vi "Main.vi"() -> ()   [LabVIEW 2016]
doc: "Main controller to read from an EK-P4 board connected to a squeezable ball, detect squeeze and release, and send it over a TCP connection to a waiting client (in this case the Matlab experiment). Choose the data file name, port and measurment interval and press start to start acquiring data. Close window to exit.\n\nSaves all data to basename_subject_id_date_time. last row in file (time = -1111) are the thresholds used.\n\ndiagram structure\n-------------------\nevent loop: start acquisition and close window.\nhardware loop: initialize, acquire data, close. all data is sent to data analysis loop\ndata analysis loop: display, save, analyze, send and receive from TCP.\nTCP loop (TCP Kernel): TCP server, sends and receives over port 55555"
uses:
  command_cluster.ctl
  data_command_enum.ctl
  HW loop state.ctl
  LoopData.ctl
  EK-P4/EK-P4.lvclass
  DataType.ctl
  FileData.ctl
  range_cluster.ctl
  EK-P4 Global.vi
  <vilib>/Utility/file.llb/Write Delimited Spreadsheet (string).vi
  <vilib>/Utility/config.llb/Read Key (Path).vi
  <vilib>/Utility/config.llb/Write Key (Path).vi
  <vilib>/Analysis/NI_AALPro.lvlib
  <vilib>/Utility/config.llb/NI_LVConfig.lvlib
panel:
  in  "Record\nTime":u16
  out "# elements in queue":i32
  in  "minimum":dbl=20.0 caption="Measurement interval [ms]"
  in  "Squeeze 2":bool
  in  "Release 2":bool
  out "strong \nrelease threshold":dbl
  out "strong\nsqueeze threshold":dbl
  out "releases 2":u16
  out "squeezes 2":u16
  out "release 2":bool
  out "squeeze 2":bool
  out "size(s) 2":i32
  out "size(s)":i32
  in  "COM port 2":refnum<visa-resource-name> caption="COM port"
  in  "COM port 1":refnum<visa-resource-name> caption="COM port"
  in  "Subject Id":string
  in  "Base File Name":string
  in  "Folder to save to":path
  in  "Release":bool
  in  "Squeeze":bool
  out "error out":errorcluster
  in  "Start":bool
  out "release":bool
  out "squeeze":bool
  in  "threshold squeeze (Pa)":dbl=100.0 caption="Measurement interval [ms]"
  in  "width (pixels)":u16=20 caption="Measurement interval [ms]"
  in  "threshold release (Pa)":dbl=-100.0 caption="Measurement interval [ms]"
  out "squeezes":u16
  out "releases":u16
  in  "Measurement interval [ms]":u16=2 min=2 step=1
  out "data string":string
  out "error  out":errorcluster
  out "Data flow/dp":dbl[][](graph) caption="Waveform Graph"
  out "integral":dbl[][](graph) caption="Waveform Graph"
  out "Status":string
  # "Measurement parameters"
  # "Squeeze-release"
  # "Testing & debug"
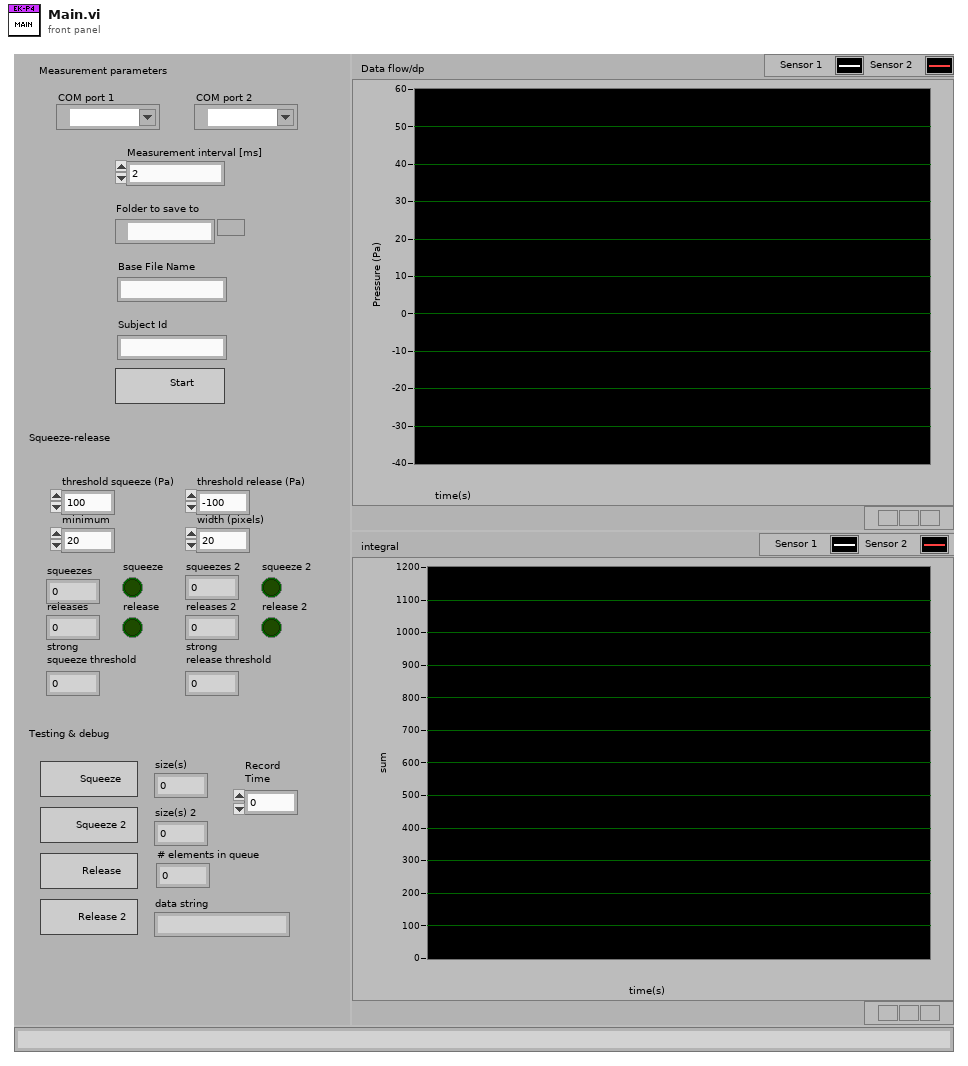
[diagram p1: front panel]
types:
  T1 = typedef "DataType.ctl" = cluster{"command":T2, "data":variant}
  T2 = typedef "data_command_enum.ctl" = enum16{"data", "display", "quit", "save", "filepath", "weak left", "state", "weak right", "strong left", "strong right", "stopRecording", "close", "sid"}
  T3 = typedef "LoopData.ctl" = cluster{"Hardware":refnum<class "EK-P4.lvclass">, "Hardware 2":refnum<class "EK-P4.lvclass">, "startTime":timestamp}
  T4 = typedef "HW loop state.ctl" = enum16{"Init", "Start", "Read", "Close", "Error", "Idle", "Exit", "Close and Exit"}
  T5 = typedef "command_cluster.ctl" = cluster{"command":T2}
  T6 = typedef "NI_LVConfig.lvlib/Config Data RefNum.ctl" = refnum<k1>
  T7 = enum16{"open", "replace", "create", "open or create", "replace or create", "replace or create with confirmation"}
  T8 = typedef "DataLoopCluster.ctl" = cluster{"all data 1":dbl[], "all data 2":dbl[], "data chunk 1":dbl[], "data chunk 2":dbl[], "number of squeezes":u16, "number of releases":u16, "Time(ms)":i64, "startWeak":timestamp, "startTime":timestamp, "Filepath":path, "time interval":u16, "recording":bool, "recording data":dbl[], "number of squeezes 2":u16, "number of releases 2":u16, "Signal":T9, "All State":string[], "Experiment State":string, "all detect state":string[], "detect State":string, "Ranges":cluster{"Strong Left":T10, "Strong Right":T10, "Weak Left":T10, "Weak Right":T10}, "ball 1":timestamp, "ball 2":timestamp, "RecordTime":u16}
  T9 = typedef "SignalType.ctl" = enum16{"weak left", "weak right", "strong left", "strong right"}
  T10 = typedef "range_cluster.ctl" = cluster{"Max":dbl, "Min":dbl}
  T11 = typedef "FileData.ctl" = cluster{"appended path":path, "Measurement interval [ms]":u16}
  T12 = enum32{"invalid app kind", "Development System", "Run Time System", "Student Edition", "Embedded LabVIEW", "Evaluation", "Custom"}
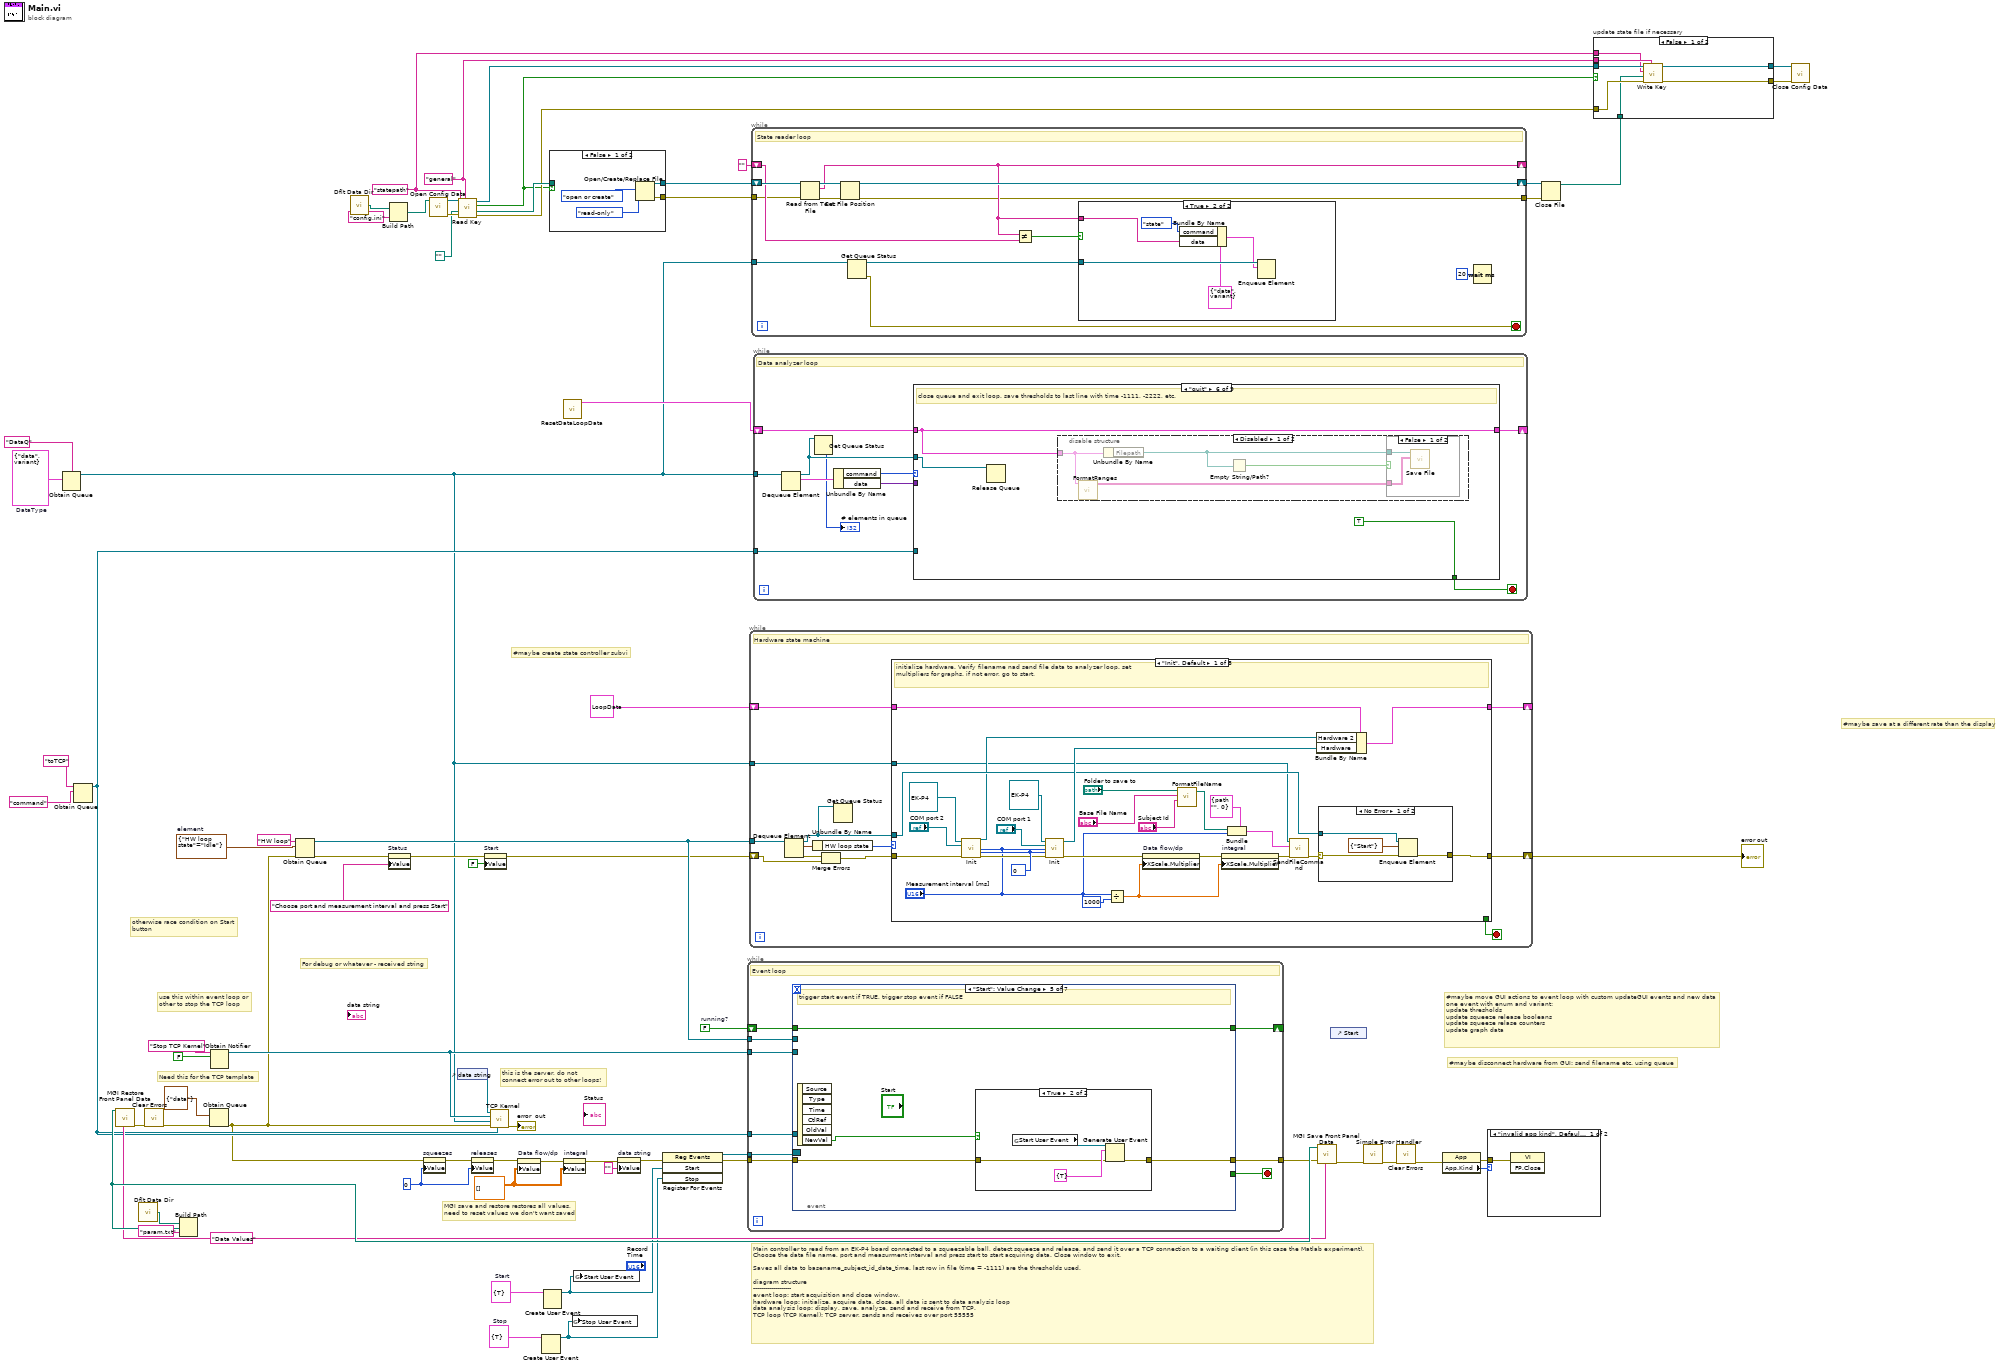
[diagram p0: block diagram]
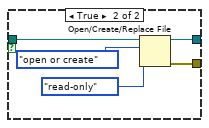
[diagram p2: hidden frame]
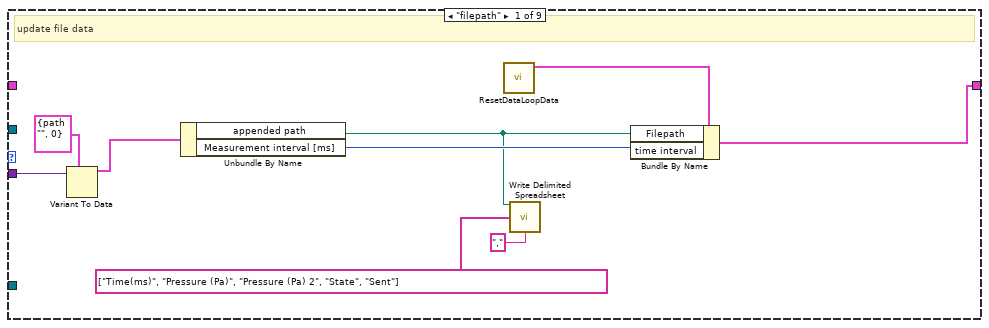
[diagram p5: hidden frame]
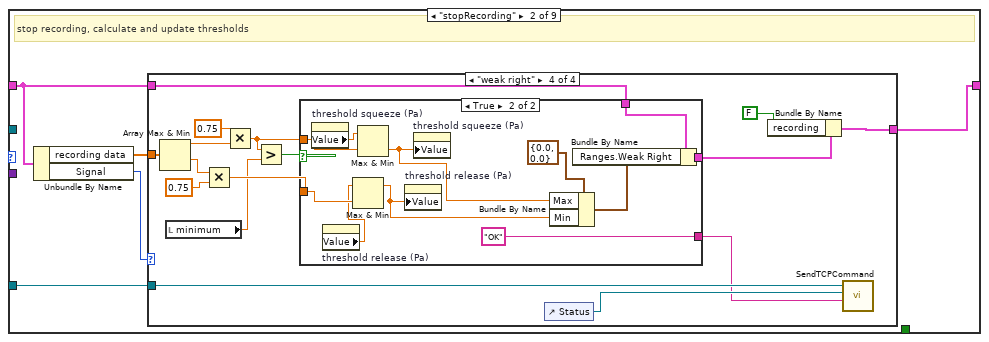
[diagram p6: hidden frame]
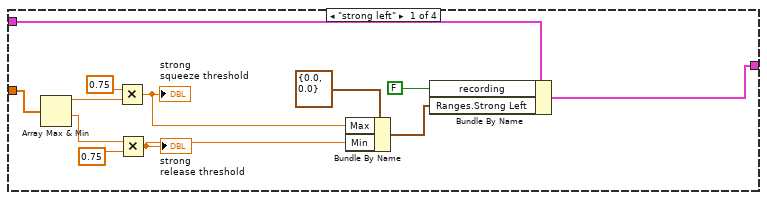
[diagram p7: hidden frame]
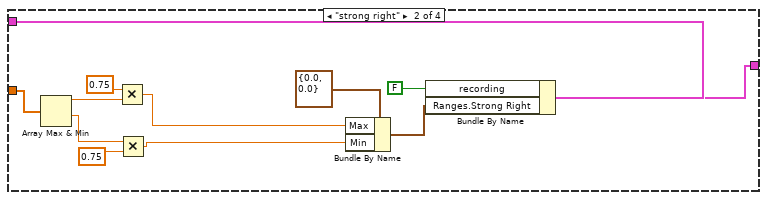
[diagram p8: hidden frame]
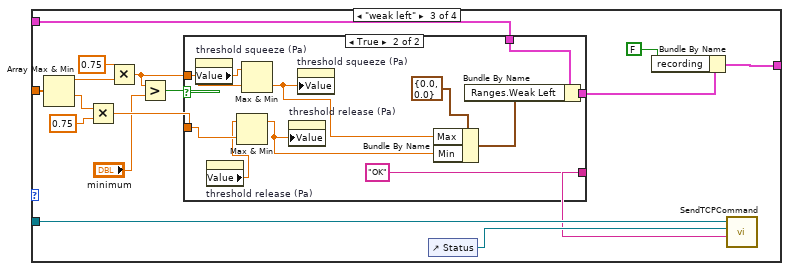
[diagram p9: hidden frame]
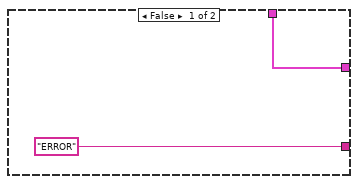
[diagram p10: hidden frame]
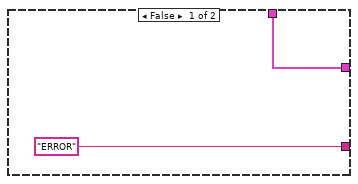
[diagram p11: hidden frame]
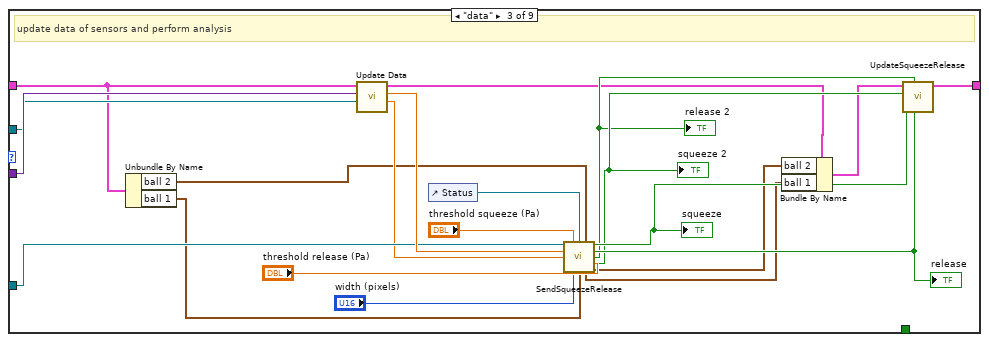
[diagram p12: hidden frame]
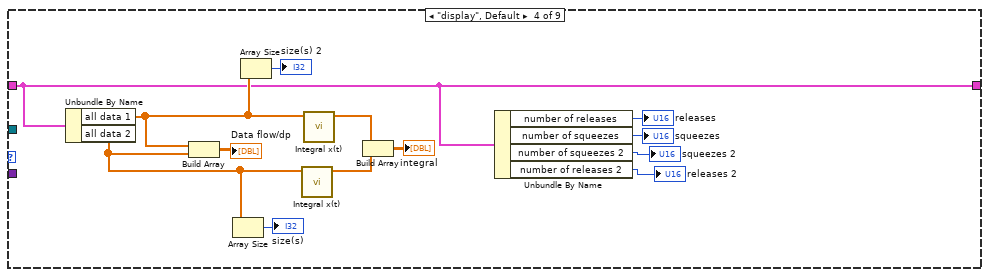
[diagram p13: hidden frame]
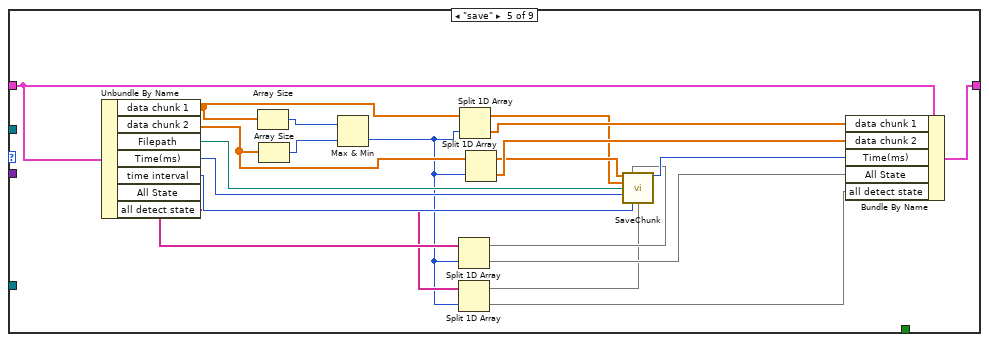
[diagram p14: hidden frame]
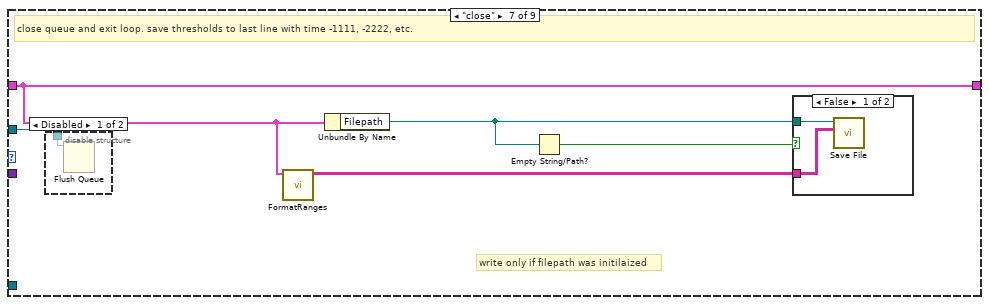
[diagram p17: hidden frame]
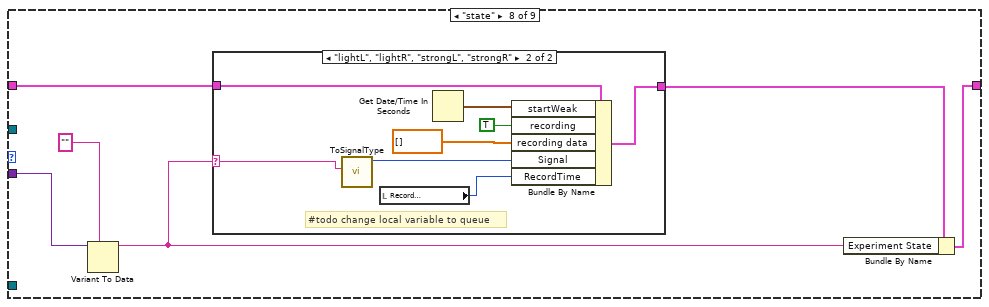
[diagram p20: hidden frame]
diagram:
  w8 = "general" ("section")
  w7 = "statepath" ("key")
  w26 = FALSE  # running?
  w28 = cluster{"Stop":bool} {"Stop"=TRUE}  # Stop
  w32 = cluster{"Start":bool} {"Start"=TRUE}  # Start
  w41 = T1 {"command"=enum."data", "data"=variant(dbl[] [])}  # DataType
  w39 = dbl[][] [] ("Data flow/dp")
  w43 = u16 0 ("squeezes")
  w49 = "Data Values" ("Section Name (\"Data Values\")")
  w62 = cluster{"HW loop state":T4} {"HW loop state"=enum."Idle"}  # element
  # "#maybe create state controller subvi"
  # "otherwise race condition on Start\nbutton"
  # "Main controller to read from an EK-P4 board connected to a squeezable ball, detect squeeze and release, and send it over a TCP connection to a waiting client (in this case the Matlab experiment). \nChoose the data file name, port and measurment interval and press start to start acquiring data. Close window to exit.\n\nSaves all data to basename_subject_id_date_time. last row in file (time = -1111) are the thresholds used.\n\ndiagram structure\n-------------------\nevent loop: start acquisition and close window.\nhardware loop: initialize, acquire data, close. all data is sent to data analysis loop\ndata analysis loop: display, save, analyze, send and receive from TCP.\nTCP loop (TCP Kernel): TCP server, sends and receives over port 55555"
  # "#maybe disconnect hardware from GUI: send filename etc. using queue"
  # "#maybe save at a different rate than the display"
  # "MGI save and restore restores all values,\nneed to reset values we don't want saved"
  # "#maybe move GUI actions to event loop with custom updateGUI events and new data\none event with enum and variant:\nupdate thresholds\nupdate squeeze release booleans\nupdate squeeze relase counters\nupdate graph data"
  # "this is the server, do not\nconnect error out to other loops!"
  # "For debug or whatever - received string"
  # "use this within event loop or \nother to stop the TCP loop"
  # "Need this for the TCP template"
  n1 = Obtain Queue(name (unnamed)="DataQ", element data type=w41) -> (queue out=w21:refnum<queue>)  [unwired: 3 in, 2 out]
  n2 = Obtain Queue(name (unnamed)="toTCP", element data type="command" ("name (unnamed)")) -> (queue out=w36:refnum<queue>)  [unwired: 3 in, 2 out]
  n3 = call <vilib>:"Dflt Data Dir.vi"() -> ("App:Default Data Directory"=w23:path)
  n4 = Build Path(base path=w23, name or relative path="param.txt") -> (appended path=w50:path)
  n5 = call <userlib>:"MGI Restore Front Panel Data.vi"("Section Name (\"Data Values\")"=w49, "Path"=w50) -> ("Error Out"=w48:errorcluster)  [unwired: 9 in]
  n6 = call <vilib>:"Clear Errors.vi"("error in (no error)"=w48) -> ("error out"=w47:errorcluster)  [unwired: 5 in, 1 out]
  n7 = Obtain Queue(element data type=T5 {"command"=enum."data"} ("chair_command_cluster"), error in (no error)=w47) -> (error out=w22:errorcluster)  [unwired: 3 in, 2 out]
  n8 = Obtain Notifier(name (unnamed)="Stop TCP Kernel", notification data type=FALSE) -> (notifier out=w64:refnum<notifier>)  [unwired: 2 in, 2 out]
  n9 = Obtain Queue(name (unnamed)="HW loop", element data type=w62, error in (no error)=w22) -> (queue out=w61:refnum<queue>, error out=w60:errorcluster)  [unwired: 2 in, 1 out]
  n10 = call <vilib>:"Dflt Data Dir.vi"() -> ("App:Default Data Directory"=w2:path)
  n11 = property on="Status" class="Str"(error in=w60, "Value"="Choose port and measurement interval and press Start" ("Status")) -> (error out=w55:errorcluster)  [unwired: 1 in, 1 out]
  n12 = Build Path(base path=w2, name or relative path="config.ini") -> (appended path=w11:path)
  n13 = property on="squeezes" class="DigNum (strict)"(error in=w22, "Value"=w43) -> (error out=w46:errorcluster)  [unwired: 1 in, 1 out]
  n14 = call <vilib>:"Open Config Data.vi"("configuration file path"=w11) -> ("error out"=w15:errorcluster, "refnum"=w14:T6)  [unwired: 8 in, 1 out]
  n15 = control-ref of="data string"() -> (w66:refnum<vi>)
  n16 = call-poly <vilib>:"Read Key.vi"("section"=w8, "error in (no error)"=w15, "default value"=path "", "key"=w7, "refnum"=w14) -> ("error out"=w6:errorcluster, "value"=w10:path, "found?"=w1:bool, "refnum out"=w9:T6)  [unwired: 3 in]
  n17 = property on="releases" class="DigNum (strict)"(error in=w46, "Value"=w43) -> (error out=w45:errorcluster)  [unwired: 1 in, 1 out]
  n18 = property on="Start" class="Bool (strict)"(error in=w55, "Value"=FALSE ("Visible")) -> (error out=w57:errorcluster)  [unwired: 1 in, 1 out]
  n19 = call "TCP Kernel.vi"("HW queue in"=w36, "error in (no error)"=w22, "queue in"=w21, "Stop Kernel Notifier"=w64, "Data indicator"=w66) -> ("error out"=→"error  out":errorcluster)  [unwired: 6 in]
  n20 = property on="Data flow/dp" class="WFGraph (strict)"(error in=w45, "Value"=w39) -> (error out=w44:errorcluster)  [unwired: 1 in, 1 out]
  n21 = Create User Event(user event datatype=w28) -> (user event=w27:refnum<user-event>)  [unwired: 1 in, 1 out]
  n22 = Create User Event(user event datatype=w32) -> (user event=w30:refnum<user-event>)  [unwired: 1 in, 1 out]
  n23 = case shown="False" w1 {
    tunnel: [w73 w80] -> w20
    tunnel: [w72 w79] -> w17
    tunnel: w10 -> [_ w76]
    frame False {
      n24 = Open/Create/Replace File(operation (0:open)=T7."open or create", access (0:read/write)=enum16{"read/write", "read-only", "write-only"}."read-only") -> (refnum out=w73:refnum<file>, error out=w72:errorcluster)  [unwired: 4 in, 1 out]
    }
    frame True {
      n25 = Open/Create/Replace File(file path (use dialog)=w76, operation (0:open)=T7."open or create", access (0:read/write)=enum16{"read/write", "read-only", "write-only"}."read-only") -> (refnum out=w80:refnum<file>, error out=w79:errorcluster)  [unwired: 3 in, 1 out]
    }
  }
  n26 = call "ResetDataLoopData.vi"() -> ("cluster"=w40:T8)  [unwired: 11 in]
  n27 = property on="integral" class="WFGraph (strict)"(error in=w44, "Value"=w39) -> (error out=w35:errorcluster)  [unwired: 1 in, 1 out]
  n28 = global write "EK-P4 Global.vi" "Stop User Event"(w27) -> ()
  n29 = global write "EK-P4 Global.vi" "Start User Event"(w30) -> ()
  n30 = property on="data string" class="Str"(error in=w35, "Value"="" ("data string")) -> (error out=w34:errorcluster)  [unwired: 1 in, 1 out]
  n31 = register-events(error in=w34, w30, w27) -> (reference out=w29:refnum<event-registration>, error out=w31:errorcluster)  [unwired: 1 in]
  n32 = while "Event loop" {
    tunnel: w64 -> [w89]
    tunnel: w31 -> [w87]
    tunnel: w61 -> [w86]
    tunnel: w36 -> [w85]
    tunnel: [w84] -> w38
    tunnel: w29 -> [w83]
    shift-right: [w81] -> _
    shift-left: w26 -> [w82]
    stop <- w88 stop-if-true
    # "Event loop"
    n33 = event shown="[4] \"Start\": Value Change" {
      selector: w83 -> [_ _ _ _ _ _ _]
      dyn-events: _ -> [_ _ _ _ _ _ _]
      timeout: _ -> [_ _ _ _ _ _ _]
      tunnel: w89 -> [_ w100 _ _ _ _ _]
      tunnel: [_ w98 _ _ _ _ _] -> w88
      tunnel: w87 -> [w91 w96 w103 w128 w146 w157 w167]
      tunnel: w86 -> [_ w97 w108 w129 _ _ _]
      tunnel: w85 -> [_ _ _ w127 _ w159 w169]
      tunnel: [w91 w96 w102 w128 w145 w157 w167] -> w84
      tunnel: w82 -> [w90 w95 w107 w126 w147 w156 w166]
      tunnel: [w90 w95 w106 w125 w147 w156 w166] -> w81
      event Timeout {
        n34 = event-data() -> ()  [unwired: 1 in, 3 out]
      }
      event Panel Close? {
        w98 = TRUE ("Discard?")
        # "exit TCP and hardware loops. If running, close and exit, otherwise exit"
        n35 = event-data() -> ()  [unwired: 1 in, 4 out]
        n36 = Send Notification(notification=TRUE, notifier=w100) -> ()  [unwired: 1 in, 2 out]
        n37 = Select(t=cluster{"HW loop state":T4} {"HW loop state"=enum."Close and Exit"}, s=w95, f=cluster{"HW loop state":T4} {"HW loop state"=enum."Exit"} ("element")) -> (s? t:f=w93:cluster{"HW loop state":T4})
        n38 = Enqueue Element(queue=w97, element=w93) -> ()  [unwired: 2 in, 3 out]
        n39 = event-data("Discard?"=w98) -> ()  [unwired: 1 in, 1 out]
      }
      event User Event {
        # "if sent with FALSE, trigger start"
        # "stop hardware acquisition and go to idle state"
        n40 = event-data() -> ("Stop"=w105:bool)  [unwired: 1 in]
        n41 = case shown="True" w107 {
          tunnel: w108 -> [_ w124]
          tunnel: [w116 FALSE ("running?")] -> w106
          tunnel: [w115 w118] -> w104
          tunnel: w103 -> [w115 w117]
          frame False {
            w116 = FALSE  # running?
          }
          frame True {
            # "go to idle state"
            n42 = control-ref of="Start"() -> (w121:refnum<vi>)
            n43 = Enqueue Element(queue=w124, element=cluster{"HW loop state":T4} {"HW loop state"=enum."Close"}, error in (no error)=w117) -> (error out=w119:errorcluster)  [unwired: 1 in, 2 out]
            n44 = property class="Bool (strict)"(reference=w121, error in=w119, "Visible"=TRUE) -> (error out=w118:errorcluster)  [unwired: 1 out]
          }
        }
        n45 = property on="Start" class="Bool (strict)"("Value"=FALSE ("Start")) -> ()  [unwired: 2 in, 2 out]
        n46 = case shown="False" w105 {
          tunnel: w104 -> [w111 w114]
          tunnel: [w110 w114] -> w102
          frame False {
            # "wait, otherwise flushes init\non close"
            n47 = global read "EK-P4 Global.vi" "Start User Event"() -> (w113:refnum<user-event>)
            n48 = Wait (ms)(milliseconds to wait=u32 500) -> ()  [unwired: 1 out]
            n49 = Generate User Event(user event=w113, event data cluster=cluster{bool} {TRUE} ("event data"), error in=w111) -> (error out=w110:errorcluster)  [unwired: 1 in, 1 out]
          }
          frame True {
          }
        }
      }
      event User Event {
        # "Start acquiring hardware data"
        n50 = event-data() -> ()  [unwired: 1 in, 5 out]
        n51 = case shown="False" w126 {
          selector: w126 -> [_ w142]
          tunnel: w129 -> [w135 _]
          tunnel: w127 -> [w132 _]
          tunnel: [TRUE ("running?") w142] -> w125
          frame False {
            # "not running - start as usual"
            n52 = disable-structure shown="Disabled" {
              disable-tunnel: w132 -> [w139 _]
              frame Disabled {
                n53 = local read "Subject Id"() -> (w137:string)
                n54 = control-ref of="Status"() -> (w140:refnum<vi>)
                n55 = Concatenate Strings("SID: " ("format string"), w137) -> (w136:string)
                n56 = call "SendTCPCommand.vi"("Command"=w136, "Status"=w140, "queue in"=w139) -> ()  [unwired: 7 in, 2 out]
              }
              frame Enabled {
              }
            }
            n57 = Enqueue Element(queue=w135, element=cluster{"HW loop state":T4} {"HW loop state"=enum."Init"}) -> ()  [unwired: 2 in, 3 out]
            n58 = property on="Status" class="Str"("Value"="Receiving data. Close window to Exit" ("Status")) -> ()  [unwired: 2 in, 2 out]
            n59 = property on="Start" class="Bool (strict)"("Value"=TRUE ("Start")) -> ()  [unwired: 2 in, 2 out]
          }
          frame True {
            # "send with false, will trigger start"
            # "already running - \nstop and start again"
            n60 = global read "EK-P4 Global.vi" "Stop User Event"() -> (w143:refnum<user-event>)
            n61 = Generate User Event(user event=w143, event data cluster=cluster{bool} {FALSE} ("event data")) -> ()  [unwired: 2 in, 2 out]
          }
        }
      }
      event "Start": Value Change {
        # "trigger start event if TRUE, trigger stop event if FALSE"
        n62 = event-data() -> ("NewVal"=w144:bool)  [unwired: 1 in, 5 out]
        n63 = case shown="True" w144 {
          tunnel: w146 -> [w149 w153]
          tunnel: [w148 w152] -> w145
          frame False {
            n64 = global read "EK-P4 Global.vi" "Stop User Event"() -> (w151:refnum<user-event>)
            n65 = Generate User Event(user event=w151, event data cluster=cluster{bool} {TRUE} ("event data"), error in=w149) -> (error out=w148:errorcluster)  [unwired: 1 in, 1 out]
          }
          frame True {
            n66 = global read "EK-P4 Global.vi" "Start User Event"() -> (w155:refnum<user-event>)
            n67 = Generate User Event(user event=w155, event data cluster=cluster{bool} {TRUE} ("event data"), error in=w153) -> (error out=w152:errorcluster)  [unwired: 1 in, 1 out]
          }
        }
      }
      event "Squeeze", "Release": Value Change {
        # "for debug, send squeeze or release over TCP"
        n68 = event-data() -> ("CtlRef"=w164:refnum<vi>)  [unwired: 1 in]
        n69 = control-ref of="Squeeze"() -> (w165:refnum<vi>)
        n70 = Equal?(x=w165, y=w164) -> (x = y?=w163:bool)
        n71 = control-ref of="Status"() -> (w158:refnum<vi>)
        n72 = Select(t="s1" ("element"), s=w163, f="r1" ("element")) -> (s? t:f=w160:string)
        n73 = call "SendTCPCommand.vi"("Command"=w160, "Status"=w158, "queue in"=w159) -> ()  [unwired: 7 in, 2 out]
      }
      event "Release 2", "Squeeze 2": Value Change {
        # "for debug, send squeeze or release over TCP"
        n74 = event-data() -> ("CtlRef"=w174:refnum<vi>)  [unwired: 1 in, 1 out]
        n75 = control-ref of="Squeeze 2"() -> (w175:refnum<vi>)
        n76 = Equal?(x=w175, y=w174) -> (x = y?=w173:bool)
        n77 = control-ref of="Status"() -> (w168:refnum<vi>)
        n78 = Select(t="s2" ("element"), s=w173, f="r2" ("element")) -> (s? t:f=w170:string)
        n79 = call "SendTCPCommand.vi"("Command"=w170, "Status"=w168, "queue in"=w169) -> ()  [unwired: 7 in, 2 out]
      }
    }
  }
  n80 = while {
    tunnel: w61 -> [w187]
    shift-right: [w183] -> _
    shift-left: T3 {"Hardware"=refnum, "Hardware 2"=refnum, "startTime"=timestamp(0 s since 1904-01-01)} ("output cluster") -> [w184]
    shift-right: [w180] -> w59
    shift-left: w57 -> [w178]
    tunnel: w21 -> [w177]
    stop <- w181 stop-if-true
    # "Hardware state machine"
    n81 = Dequeue Element(queue=w187) -> (queue out=w176:refnum<queue>, element=w186:cluster{"HW loop state":T4}, error out=w182:errorcluster)  [unwired: 2 in, 1 out]
    n82 = Unbundle By Name(w186) -> ("HW loop state"=w185:T4)
    n83 = Merge Errors(w182, w178) -> (w179:errorcluster)
    n84 = Get Queue Status(queue=w176) -> ()  [unwired: 2 in, 8 out]
    n85 = case shown="\"Init\", Default" w185 {
      tunnel: w184 -> [w205 w231 w259 w288 w303 w312 w323 w330]
      tunnel: [w213 w230 w259 w288 w303 w312 w323 w330] -> w183
      tunnel: w176 -> [w206 w225 w260 w279 _ _ w319 w328]
      tunnel: w179 -> [w198 w235 w263 w285 w301 w309 w322 w329]
      tunnel: [w207 w227 w261 w280 w301 w305 w316 w325] -> w180
      tunnel: [_ _ _ FALSE TRUE TRUE _ _] -> w181
      tunnel: w177 -> [w195 _ w257 w282 w300 w306 _ _]
      frame "Init", Default {
        w200 = u8 0 ("address (USB SensorCable) 2")
        # "initialize hardware. Verify filename nad send file data to analyzer loop. set\nmultipliers for graphs. if not error, go to start."
        n86 = call-dynamic "Init.vi"("EK-P4.lvclass"=refnum<class "EK-P4.lvclass"> refnum, "VISA Refnum in"="COM port 2", "Measurement interval [ms] in"="Measurement interval [ms]", "address (USB SensorCable)"=w200, "error in (no error)"=w198) -> ("EK-P4.lvclass 2"=w199:refnum<class "EK-P4.lvclass">, "error out"=w197:errorcluster)  [unwired: 8 in, 1 out]
        n87 = call-dynamic "Init.vi"("EK-P4.lvclass"=refnum<class "EK-P4.lvclass"> refnum, "VISA Refnum in"="COM port 1", "Measurement interval [ms] in"="Measurement interval [ms]", "address (USB SensorCable)"=w200, "error in (no error)"=w197) -> ("EK-P4.lvclass 2"=w209:refnum<class "EK-P4.lvclass">, "error out"=w196:errorcluster)  [unwired: 8 in, 1 out]
        n88 = Divide(x="Measurement interval [ms]", y=u16 1000) -> (x/y=w211:dbl)
        n89 = property on="Data flow/dp" class="WFGraph (strict)"(error in=w196, "XScale.Multiplier"=w211) -> (error out=w208:errorcluster)  [unwired: 1 in, 1 out]
        n90 = call "FormatFileName.vi"("Subject Id"="Subject Id", "Base file Name"="Base File Name", "Folder to save to"="Folder to save to") -> ("appended path"=w192:path)  [unwired: 8 in]
        n91 = property on="integral" class="WFGraph (strict)"(error in=w208, "XScale.Multiplier"=w211) -> (error out=w194:errorcluster)  [unwired: 1 in, 1 out]
        n92 = Bundle(cluster=T11 {"appended path"=path "", "Measurement interval [ms]"=0}, "appended path"=w192, "Measurement interval [ms]"="Measurement interval [ms]") -> (w190:T11)
        n93 = call "SendFileCommand.vi"("error in (no error)"=w194, "file data"=w190, "Queue in"=w195) -> ("error out"=w193:errorcluster)  [unwired: 7 in, 1 out]
        n94 = Bundle By Name(cluster=w205, "Hardware 2"=w199, "Hardware"=w209) -> (w213:T3)
        n95 = case shown="No Error" w193 {
          selector: w193 -> [w217 w219]
          tunnel: [w216 w221] -> w207
          tunnel: w206 -> [w215 w222]
          frame No Error {
            n96 = Enqueue Element(queue=w215, element=cluster{"HW loop state":T4} {"HW loop state"=enum."Start"}, error in (no error)=w217) -> (error out=w216:errorcluster)  [unwired: 1 in, 2 out]
          }
          frame Error {
            n97 = Enqueue Element(queue=w222, element=cluster{"HW loop state":T4} {"HW loop state"=enum."Error"}) -> (error out=w220:errorcluster)  [unwired: 2 in, 2 out]
            n98 = Merge Errors(w220, w219) -> (w221:errorcluster)
          }
        }
      }
      frame "Start" {
        # "if not error go to read"
        # "start measurement in each sensor. Becasue they can't be started exactly simulataneously, the sensors have a small phase difference. this is ignored in the file and everywhere else. save start time for timing of display and save commands"
        n99 = Unbundle By Name(w231) -> ("Hardware 2"=w232:refnum<class "EK-P4.lvclass">, "Hardware"=w233:refnum<class "EK-P4.lvclass">)
        n100 = call-dynamic "Start Measurement.vi"("EK-P4.lvclass"=w233, "error in (no error)"=w235) -> ("EK-P4.lvclass 2"=w228:refnum<class "EK-P4.lvclass">, "error out"=w234:errorcluster)  [unwired: 12 in]
        n101 = call-dynamic "Start Measurement.vi"("EK-P4.lvclass"=w232, "error in (no error)"=w234) -> ("EK-P4.lvclass 2"=w229:refnum<class "EK-P4.lvclass">, "error out"=w226:errorcluster)  [unwired: 12 in]
        n102 = Get Date/Time In Seconds() -> (seconds since 1Jan1904=w224:timestamp)
        n103 = case shown="No Error" w226 {
          selector: w226 -> [w238 w240]
          tunnel: [w237 w242] -> w227
          tunnel: w225 -> [w236 w243]
          frame No Error {
            n104 = Enqueue Element(queue=w236, element=cluster{"HW loop state":T4} {"HW loop state"=enum."Read"}, error in (no error)=w238) -> (error out=w237:errorcluster)  [unwired: 1 in, 2 out]
          }
          frame Error {
            n105 = Enqueue Element(queue=w243, element=cluster{"HW loop state":T4} {"HW loop state"=enum."Error"}) -> (error out=w241:errorcluster)  [unwired: 2 in, 2 out]
            n106 = Merge Errors(w241, w240) -> (w242:errorcluster)
          }
        }
        n107 = Bundle By Name(cluster=w231, "Hardware 2"=w229, "Hardware"=w228, "startTime"=w224) -> (w230:T3)
      }
      frame "Read" {
        # "display and save according to display rate"
        # "read and send data. If time for it, send display and save commands as well. if not error, continue reading"
        n108 = Unbundle By Name(w259) -> ("Hardware 2"=w258:refnum<class "EK-P4.lvclass">, "Hardware"=w262:refnum<class "EK-P4.lvclass">)
        n109 = Unbundle By Name(w259) -> ("startTime"=w250:timestamp)
        n110 = call-dynamic "Read Data.vi"("EK-P4 in"=w258) -> ("error out"=w254:errorcluster, "Data"=w247:dbl[])  [unwired: 6 in, 3 out]
        n111 = call-dynamic "Read Data.vi"("error in (no error)"=w263, "EK-P4 in"=w262) -> ("error out"=w255:errorcluster, "Data"=w246:dbl[])  [unwired: 5 in, 3 out]
        n112 = call "updateRate.vi"("display rate"=0.3, "startTime"=w250) -> ("Boolean"=w249:bool)  [unwired: 9 in]
        n113 = Wait (ms)(milliseconds to wait=u32 50) -> ()  [unwired: 1 out]
        n114 = Merge Errors(w254, w255) -> (w253:errorcluster)
        n115 = call "SendDataCommand.vi"("error in (no error)"=w253, "Data 2"=w247, "Data"=w246, "Queue in"=w257) -> ("error out"=w252:errorcluster, "Queue out"=w256:refnum<queue>)  [unwired: 6 in]
        n116 = case shown="True" w249 {
          tunnel: w256 -> [_ w269]
          tunnel: w252 -> [w264 w268]
          tunnel: [w264 w265] -> w251
          frame False {
          }
          frame True {
            n117 = call "SendDisplayCommand.vi"("error in (no error)"=w268, "Queue in"=w269) -> ("error out"=w266:errorcluster, "queue out"=w267:refnum<queue>)  [unwired: 8 in]
            n118 = call "SendSaveCommand.vi"("error in (no error)"=w266, "Queue in"=w267) -> ("error out"=w265:errorcluster)  [unwired: 8 in, 1 out]
          }
        }
        n119 = case shown="No Error" w251 {
          selector: w251 -> [w272 w274]
          tunnel: [w271 w275] -> w261
          tunnel: w260 -> [w270 w276]
          frame No Error {
            n120 = Enqueue Element(queue=w270, element=cluster{"HW loop state":T4} {"HW loop state"=enum."Read"}, error in (no error)=w272) -> (error out=w271:errorcluster)  [unwired: 1 in, 2 out]
          }
          frame Error {
            n121 = Enqueue Element(queue=w276, element=cluster{"HW loop state":T4} {"HW loop state"=enum."Error"}) -> (error out=w277:errorcluster)  [unwired: 2 in, 2 out]
            n122 = Merge Errors(w277, w274) -> (w275:errorcluster)
          }
        }
      }
      frame "Close" {
        # "close hardware and send quit to data analyzer loop. exit loop"
        n123 = Unbundle By Name(w288) -> ("Hardware 2"=w284:refnum<class "EK-P4.lvclass">, "Hardware"=w286:refnum<class "EK-P4.lvclass">)
        n124 = call "SendCloseCommand.vi"("Queue in"=w282) -> ()  [unwired: 9 in, 2 out]
        n125 = call-dynamic "Close.vi"("error in (no error)"=w285, "EK-P4 in"=w286) -> ("error out"=w283:errorcluster)  [unwired: 8 in, 1 out]
        n126 = call-dynamic "Close.vi"("error in (no error)"=w283, "EK-P4 in"=w284) -> ("error out"=w281:errorcluster)  [unwired: 8 in, 1 out]
        n127 = case shown="No Error" w281 {
          selector: w281 -> [w290 w295]
          tunnel: [w293 w296] -> w280
          tunnel: w279 -> [w292 w297]
          frame No Error {
            n128 = Flush Queue(queue=w292, error in (no error)=w290) -> (queue out=w291:refnum<queue>, error out=w289:errorcluster)  [unwired: 1 out]
            n129 = Enqueue Element(queue=w291, element=cluster{"HW loop state":T4} {"HW loop state"=enum."Idle"}, error in (no error)=w289) -> (error out=w293:errorcluster)  [unwired: 1 in, 2 out]
          }
          frame Error {
            n130 = Enqueue Element(queue=w297, element=cluster{"HW loop state":T4} {"HW loop state"=enum."Error"}) -> (error out=w298:errorcluster)  [unwired: 2 in, 2 out]
            n131 = Merge Errors(w298, w295) -> (w296:errorcluster)
          }
        }
      }
      frame "Exit" {
        # "close hardware and send quit to data analyzer loop. exit loop"
        n132 = disable-structure shown="Enabled" {
          disable-tunnel: w300 -> [w304 _]
          frame Enabled {
            n133 = call "SendQuitCommand.vi"("Queue in"=w304) -> ()  [unwired: 9 in, 2 out]
          }
          frame Disabled {
          }
        }
      }
      frame "Close and Exit" {
        # "close hardware and send quit to data analyzer loop. exit loop"
        n134 = disable-structure shown="Enabled" {
          disable-tunnel: w306 -> [w314 _]
          frame Enabled {
            n135 = call "SendCloseCommand.vi"("Queue in"=w314) -> ("queue out"=w313:refnum<queue>)  [unwired: 9 in, 1 out]
            n136 = call "SendQuitCommand.vi"("Queue in"=w313) -> ()  [unwired: 9 in, 2 out]
          }
          frame Disabled {
          }
        }
        n137 = Unbundle By Name(w312) -> ("Hardware 2"=w308:refnum<class "EK-P4.lvclass">, "Hardware"=w310:refnum<class "EK-P4.lvclass">)
        n138 = call-dynamic "Close.vi"("error in (no error)"=w309, "EK-P4 in"=w310) -> ("error out"=w307:errorcluster)  [unwired: 8 in, 1 out]
        n139 = call-dynamic "Close.vi"("error in (no error)"=w307, "EK-P4 in"=w308) -> ("error out"=w305:errorcluster)  [unwired: 8 in, 1 out]
      }
      frame "Error" {
        # "basic error handling: show error, clear error, exit."
        n140 = call <vilib>:"Simple Error Handler.vi"("error in (no error)"=w322) -> ("error out"=w321:errorcluster)  [unwired: 4 in, 4 out]
        n141 = call <vilib>:"Clear Errors.vi"("error in (no error)"=w321) -> ("error out"=w318:errorcluster)  [unwired: 5 in, 1 out]
        n142 = Enqueue Element(queue=w319, element=cluster{"HW loop state":T4} {"HW loop state"=enum."Exit"}, error in (no error)=w318) -> (error out=w317:errorcluster)  [unwired: 1 in, 2 out]
        n143 = property on="Status" class="Str"(error in=w317, "Value"="Error communicating with Ek-P4, closing connection. Close window to exit." ("Status")) -> (error out=w316:errorcluster)  [unwired: 1 in, 1 out]
      }
      frame "Idle" {
        # "do nothing"
        n144 = Wait (ms)(milliseconds to wait=u32 200) -> ()  [unwired: 1 out]
        n145 = disable-structure shown="Enabled" {
          disable-tunnel: w329 -> [w334 w335]
          disable-tunnel: w328 -> [w332 _]
          disable-tunnel: [w331 w335] -> w326
          frame Disabled {
            n146 = Enqueue Element(queue=w332, element=cluster{"HW loop state":T4} {"HW loop state"=enum."Idle"}, error in (no error)=w334) -> (error out=w331:errorcluster)  [unwired: 1 in, 2 out]
          }
          frame Enabled {
          }
        }
        n147 = property on="Status" class="Str"(error in=w326, "Value"="waiting for client..." ("Status")) -> (error out=w325:errorcluster)  [unwired: 1 in, 1 out]
      }
    }
  }
  "error out" <- w59
  n148 = while {
    tunnel: w21 -> [w343]
    shift-right: [w346] -> w19
    shift-left: w20 -> [w348]
    shift-right: [w342] -> _
    shift-left: "" -> [w345]
    tunnel: w17 -> [w339]
    tunnel: [w337] -> w16
    stop <- w340 stop-if-true
    # "State reader loop"
    n149 = Read from Text File(file (use dialog)=w348, error in=w339) -> (refnum out=w347:refnum<file>, text=w342:string, error out=w338:errorcluster)  [unwired: 2 in, 1 out]
    n150 = Set File Position(refnum=w347, error in=w338) -> (refnum out=w346:refnum<file>, error out=w337:errorcluster)  [unwired: 2 in]
    n151 = Get Queue Status(queue=w343) -> (queue out=w341:refnum<queue>, error out=w340:errorcluster)  [unwired: 2 in, 6 out]
    n152 = Not Equal?(x=w342, y=w345) -> (x != y?=w344:bool)
    n153 = case shown="True" w344 {
      tunnel: w341 -> [_ w353]
      tunnel: w342 -> [_ w350]
      frame False {
      }
      frame True {
        n154 = Bundle By Name(cluster=T1 {"command"=enum."data", "data"=variant} ("element"), "command"=data_command_enum."state", "data"=w350) -> (w349:T1)
        n155 = Enqueue Element(queue=w353, element=w349) -> ()  [unwired: 2 in, 3 out]
      }
    }
    n156 = Wait (ms)(milliseconds to wait=u32 20) -> ()  [unwired: 1 out]
  }
  n157 = while {
    tunnel: w21 -> [w363]
    shift-right: [w358] -> _
    shift-left: w40 -> [w359]
    tunnel: w36 -> [w356]
    stop <- w360 stop-if-true
    # "Data analyzer loop"
    n158 = Dequeue Element(queue=w363) -> (queue out=w355:refnum<queue>, element=w362:T1)  [unwired: 2 in, 2 out]
    n159 = Get Queue Status(queue=w355) -> (# elements in queue=→"# elements in queue":i32)  [unwired: 2 in, 7 out]
    n160 = Unbundle By Name(w362) -> ("command"=w361:T2, "data"=w357:variant)
    n161 = case shown="\"quit\"" w361 {
      tunnel: [_ _ _ _ _ TRUE _ _ _] -> w360
      tunnel: w359 -> [_ w377 w466 w483 w511 w515 w524 w534 w548]
      tunnel: [w371 w376 w473 w483 w510 w515 w524 w536 w548] -> w358
      tunnel: w357 -> [w372 _ w480 _ _ _ _ w537 w550]
      tunnel: w355 -> [_ _ w470 _ _ w516 w525 _ _]
      tunnel: w356 -> [_ w374 w474 _ _ _ _ _ _]
      frame "filepath" {
        # "update file data"
        n162 = Variant To Data(type=T11 {"appended path"=path "", "Measurement interval [ms]"=0} ("cluster"), Variant=w372) -> (data=w369:T11)  [unwired: 1 in, 1 out]
        n163 = Unbundle By Name(w369) -> ("appended path"=w367:path, "Measurement interval [ms]"=w368:u16)
        n164 = call "ResetDataLoopData.vi"() -> ("cluster"=w364:T8)  [unwired: 11 in]
        n165 = call-poly <vilib>:"Write Delimited Spreadsheet.vi"("file path (dialog if empty)"=w367, "1D data"=string[] ["Time(ms)", "Pressure (Pa)", "Pressure (Pa) 2", "State", "Sent"] ("Header Lines[row][col]"), "delimiter (\\t)"="," ("delimiter (\\t)")) -> ()  [unwired: 11 in, 2 out]
        n166 = Bundle By Name(cluster=w364, "Filepath"=w367, "time interval"=w368) -> (w371:T8)
      }
      frame "stopRecording" {
        # "stop recording, calculate and update thresholds"
        n167 = Unbundle By Name(w377) -> ("recording data"=w375:dbl[], "Signal"=w373:T9)
        n168 = case shown="\"weak right\"" w373 {
          tunnel: w377 -> [w388 w400 w403 w433]
          tunnel: [w387 w399 w417 w446] -> w376
          tunnel: w375 -> [w382 w394 w415 w444]
          tunnel: w374 -> [_ _ w406 w436]
          frame "strong left" {
            n169 = Array Max & Min(array=w382) -> (max value=w386:dbl, min value=w384:dbl)  [unwired: 2 out]
            n170 = Multiply(x=0.75, y=w386) -> (x*y=w381:dbl)
            "strong\nsqueeze threshold" <- w381
            n171 = Multiply(x=w384, y=0.75 ("x")) -> (x*y=w380:dbl)
            "strong \nrelease threshold" <- w380
            n172 = Bundle By Name(cluster=T10 {"Max"=0.0, "Min"=0.0} ("Ranges.Strong Left"), "Max"=w381, "Min"=w380) -> (w378:T10)
            n173 = Bundle By Name(cluster=w388, "recording"=FALSE, "Ranges.Strong Left"=w378) -> (w387:T8)
          }
          frame "strong right" {
            n174 = Array Max & Min(array=w394) -> (max value=w398:dbl, min value=w396:dbl)  [unwired: 2 out]
            n175 = Multiply(x=0.75, y=w398) -> (x*y=w393:dbl)
            n176 = Multiply(x=w396, y=0.75 ("x")) -> (x*y=w392:dbl)
            n177 = Bundle By Name(cluster=T10 {"Max"=0.0, "Min"=0.0} ("Ranges.Strong Left"), "Max"=w393, "Min"=w392) -> (w390:T10)
            n178 = Bundle By Name(cluster=w400, "recording"=FALSE, "Ranges.Strong Right"=w390) -> (w399:T8)
          }
          frame "weak left" {
            n179 = Array Max & Min(array=w415) -> (max value=w414:dbl, min value=w412:dbl)  [unwired: 2 out]
            n180 = Multiply(x=w412, y=0.75 ("x")) -> (x*y=w410:dbl)
            n181 = Multiply(x=0.75, y=w414) -> (x*y=w409:dbl)
            n182 = Greater?(x=w409, y="minimum") -> (0:w407:bool)
            n183 = case shown="True" w407 {
              tunnel: w409 -> [_ w430]
              tunnel: w410 -> [_ w429]
              tunnel: ["ERROR" "OK"] -> w404
              tunnel: w403 -> [w418 w424]
              tunnel: [w418 w422] -> w402
              frame False {
              }
              frame True {
                n184 = property on="threshold squeeze (Pa)" class="DigNum (strict)"() -> ("Value"=w426:dbl)  [unwired: 2 in, 2 out]
                n185 = property on="threshold release (Pa)" class="DigNum (strict)"() -> ("Value"=w427:dbl)  [unwired: 2 in, 2 out]
                n186 = Max & Min(x=w427, y=w429) -> (max(x,y)=w420:dbl)  [unwired: 1 out]
                n187 = Max & Min(x=w426, y=w430) -> (min(x,y)=w421:dbl)  [unwired: 1 out]
                n188 = property on="threshold release (Pa)" class="DigNum (strict)"("Value"=w420) -> ()  [unwired: 2 in, 2 out]
                n189 = property on="threshold squeeze (Pa)" class="DigNum (strict)"("Value"=w421) -> ()  [unwired: 2 in, 2 out]
                n190 = Bundle By Name(cluster=T10 {"Max"=0.0, "Min"=0.0} ("Ranges.Weak Left"), "Max"=w421, "Min"=w420) -> (w423:T10)
                n191 = Bundle By Name(cluster=w424, "Ranges.Weak Left"=w423) -> (w422:T8)
              }
            }
            n192 = control-ref of="Status"() -> (w405:refnum<vi>)
            n193 = Bundle By Name(cluster=w402, "recording"=FALSE) -> (w417:T8)
            n194 = call "SendTCPCommand.vi"("Command"=w404, "Status"=w405, "queue in"=w406) -> ()  [unwired: 7 in, 2 out]
          }
          frame "weak right" {
            n195 = Array Max & Min(array=w444) -> (max value=w443:dbl, min value=w441:dbl)  [unwired: 2 out]
            n196 = local read "minimum"() -> (w431:dbl)
            n197 = Multiply(x=w441, y=0.75 ("x")) -> (x*y=w439:dbl)
            n198 = Multiply(x=0.75, y=w443) -> (x*y=w438:dbl)
            n199 = Greater?(x=w438, y=w431) -> (0:w437:bool)
            n200 = case shown="True" w437 {
              tunnel: w438 -> [_ w459]
              tunnel: w439 -> [_ w458]
              tunnel: ["ERROR" "OK"] -> w434
              tunnel: w433 -> [w447 w453]
              tunnel: [w447 w451] -> w432
              frame False {
              }
              frame True {
                n201 = property on="threshold squeeze (Pa)" class="DigNum (strict)"() -> ("Value"=w455:dbl)  [unwired: 2 in, 2 out]
                n202 = property on="threshold release (Pa)" class="DigNum (strict)"() -> ("Value"=w456:dbl)  [unwired: 2 in, 2 out]
                n203 = Max & Min(x=w456, y=w458) -> (max(x,y)=w449:dbl)  [unwired: 1 out]
                n204 = Max & Min(x=w455, y=w459) -> (min(x,y)=w450:dbl)  [unwired: 1 out]
                n205 = property on="threshold release (Pa)" class="DigNum (strict)"("Value"=w449) -> ()  [unwired: 2 in, 2 out]
                n206 = property on="threshold squeeze (Pa)" class="DigNum (strict)"("Value"=w450) -> ()  [unwired: 2 in, 2 out]
                n207 = Bundle By Name(cluster=T10 {"Max"=0.0, "Min"=0.0} ("Ranges.Weak Left"), "Max"=w450, "Min"=w449) -> (w452:T10)
                n208 = Bundle By Name(cluster=w453, "Ranges.Weak Right"=w452) -> (w451:T8)
              }
            }
            n209 = control-ref of="Status"() -> (w435:refnum<vi>)
            n210 = Bundle By Name(cluster=w432, "recording"=FALSE) -> (w446:T8)
            n211 = call "SendTCPCommand.vi"("Command"=w434, "Status"=w435, "queue in"=w436) -> ()  [unwired: 7 in, 2 out]
          }
        }
      }
      frame "data" {
        # "update data of sensors and perform analysis"
        n212 = Unbundle By Name(w466) -> ("ball 2"=w465:timestamp, "ball 1"=w461:timestamp)
        n213 = call "Update Data.vi"("queue out"=w470, "data"=w480, "cluster in"=w466) -> ("data element  2"=w469:dbl, "data element  1"=w476:dbl, "cluster out"=w464:T8)  [unwired: 6 in]
        n214 = control-ref of="Status"() -> (w479:refnum<vi>)
        n215 = call "SendSqueezeRelease.vi"("Queue in"=w474, "threshold squeeze in"="threshold squeeze (Pa)", "Status"=w479, "ball 2"=w465, "data 1"=w476, "data2"=w469, "threshold release in"="threshold release (Pa)", "width squeeze in"="width (pixels)", "ball 1"=w461) -> ("peak"=w472:bool, "valley"=w471:bool, "valley 2"=w467:bool, "peak 2"=w468:bool, "ball 1 out"=w460:timestamp, "ball 2 out"=w462:timestamp)  [unwired: 1 in]
        "release" <- w471
        "squeeze" <- w472
        "squeeze 2" <- w468
        "release 2" <- w467
        n216 = Bundle By Name(cluster=w464, "ball 2"=w462, "ball 1"=w460) -> (w463:T8)
        n217 = call "UpdateSqueezeRelease.vi"("valley"=w471, "valley 2"=w467, "peak"=w472, "peak 2"=w468, "Loop Data"=w463) -> ("DataLoop"=w473:T8)  [unwired: 6 in]
      }
      frame "display", Default {
        n218 = Unbundle By Name(w483) -> ("all data 1"=w488:dbl[], "all data 2"=w484:dbl[])
        n219 = Build Array(w488, w484) -> (→"Data flow/dp":dbl[][])
        n220 = Array Size(array=w484) -> (size(s)=→"size(s)":i32)
        n221 = Array Size(array=w488) -> (size(s)=→"size(s) 2":i32)
        n222 = call <vilib>:"Integral x(t).vi"("X"=w484) -> ("Integral X"=w491:dbl[])  [unwired: 9 in, 1 out]
        n223 = call <vilib>:"Integral x(t).vi"("X"=w488) -> ("Integral X"=w492:dbl[])  [unwired: 9 in, 1 out]
        n224 = Build Array(w492, w491) -> (→"integral":dbl[][])
        n225 = Unbundle By Name(w483) -> ("number of releases"=→"releases":u16, "number of squeezes"=→"squeezes":u16, "number of squeezes 2"=→"squeezes 2":u16, "number of releases 2"=→"releases 2":u16)
      }
      frame "save" {
        n226 = Unbundle By Name(w511) -> ("data chunk 1"=w512:dbl[], "data chunk 2"=w506:dbl[], "Filepath"=w502:path, "Time(ms)"=w507:i64, "time interval"=w501:u16, "All State"=w500:string[], "all detect state"=w497:string[])
        n227 = Array Size(array=w512) -> (size(s)=w514:i32)
        n228 = Array Size(array=w506) -> (size(s)=w513:i32)
        n229 = Max & Min(x=w514, y=w513) -> (min(x,y)=w496:i32)  [unwired: 1 out]
        n230 = Split 1D Array(array=w500, index=w496) -> (first subarray=w499:string[], second subarray=w498:string[])
        n231 = Split 1D Array(array=w497, index=w496) -> (first subarray=w494:string[], second subarray=w495:string[])
        n232 = Split 1D Array(array=w512, index=w496) -> (first subarray=w503:dbl[], second subarray=w509:dbl[])
        n233 = Split 1D Array(array=w506, index=w496) -> (first subarray=w504:dbl[], second subarray=w508:dbl[])
        n234 = call "SaveChunk.vi"("Sensor2"=w504, "All State"=w499, "Sensor1"=w503, "Path"=w502, "Time(ms)"=w507, "Time interval"=w501, "all detect"=w494) -> ("Time (ms) out"=w505:i64)  [unwired: 7 in, 1 out]
        n235 = Bundle By Name(cluster=w511, "data chunk 1"=w509, "data chunk 2"=w508, "Time(ms)"=w505, "All State"=w498, "all detect state"=w495) -> (w510:T8)
      }
      frame "quit" {
        # "close queue and exit loop. save thresholds to last line with time -1111, -2222, etc."
        n236 = Release Queue(queue=w516) -> ()  [unwired: 2 in, 3 out]
        n237 = disable-structure shown="Disabled" {
          disable-tunnel: w515 -> [w518 _]
          frame Disabled {
            n238 = call "FormatRanges.vi"("cluster"=w518) -> ("range string array"=w521:string[][])  [unwired: 10 in]
            n239 = Unbundle By Name(w518) -> ("Filepath"=w520:path)
            n240 = Empty String/Path?(string/path=w520) -> (empty?=w519:bool)
            n241 = case shown="False" w519 {
              tunnel: w521 -> [w523 _]
              tunnel: w520 -> [w522 _]
              frame False {
                n242 = call "Save File.vi"("Array"=w523, "Path"=w522) -> ()  [unwired: 9 in, 1 out]
              }
              frame True {
              }
            }
          }
          frame Enabled {
          }
        }
      }
      frame "close" {
        # "write only if filepath was initilaized"
        # "close queue and exit loop. save thresholds to last line with time -1111, -2222, etc."
        n243 = disable-structure shown="Disabled" {
          disable-tunnel: w525 -> [w529 _]
          frame Disabled {
            n244 = Flush Queue(queue=w529) -> ()  [unwired: 1 in, 3 out]
          }
          frame Enabled {
          }
        }
        n245 = call "FormatRanges.vi"("cluster"=w524) -> ("range string array"=w528:string[][])  [unwired: 10 in]
        n246 = Unbundle By Name(w524) -> ("Filepath"=w527:path)
        n247 = Empty String/Path?(string/path=w527) -> (empty?=w526:bool)
        n248 = case shown="False" w526 {
          tunnel: w528 -> [w531 _]
          tunnel: w527 -> [w530 _]
          frame False {
            n249 = call "Save File.vi"("Array"=w531, "Path"=w530) -> ()  [unwired: 9 in, 1 out]
          }
          frame True {
          }
        }
      }
      frame "state" {
        n250 = Variant To Data(type="" ("Experiment State"), Variant=w537) -> (data=w532:string)  [unwired: 1 in, 1 out]
        n251 = case shown="\"lightL\", \"lightR\", \"strongL\", \"strongR\"" w532 {
          selector: w532 -> [_ w540]
          tunnel: w534 -> [w538 w542]
          tunnel: [w538 w541] -> w533
          frame "False", Default {
          }
          frame "lightL", "lightR", "strongL", "strongR" {
            # "#todo change local variable to queue"
            n252 = call "ToSignalType.vi"("state"=w540) -> ("Signal"=w543:T9)  [unwired: 10 in]
            n253 = local read "Record\nTime"() -> (w539:u16)
            n254 = Get Date/Time In Seconds() -> (seconds since 1Jan1904=w545:timestamp)
            n255 = Bundle By Name(cluster=w542, "startWeak"=w545, "recording"=TRUE, "recording data"=dbl[] [], "Signal"=w543, "RecordTime"=w539) -> (w541:T8)
          }
        }
        n256 = Bundle By Name(cluster=w533, "Experiment State"=w532) -> (w536:T8)
      }
      frame "sid" {
        n257 = Variant To Data(type="" ("Experiment State"), Variant=w550) -> (data=w547:string)  [unwired: 1 in, 1 out]
        n258 = property on="Subject Id" class="Str"("Value"=w547) -> ()  [unwired: 2 in, 2 out]
      }
    }
  }
  n259 = call <userlib>:"MGI Save Front Panel Data.vi"("Section Name (\"Data Values\")"=w49, "error in (no error)"=w38, "Path"=w50) -> ("Error Out"=w37:errorcluster)  [unwired: 8 in]
  n260 = control-ref of="Start"() -> ()  [unwired: 1 out]
  n261 = call <vilib>:"Simple Error Handler.vi"("error in (no error)"=w37) -> ("error out"=w25:errorcluster)  [unwired: 4 in, 4 out]
  n262 = call <vilib>:"Clear Errors.vi"("error in (no error)"=w25) -> ("error out"=w24:errorcluster)  [unwired: 5 in, 1 out]
  n263 = property class="App"(error in=w24) -> (error out=w52:errorcluster, "App.Kind"=w53:T12)  [unwired: 1 in, 1 out]
  n264 = case shown="\"invalid app kind\", Default" w53 {
    tunnel: w52 -> [w551 _]
    frame "invalid app kind", Default {
      n265 = invoke class="VI" method="FP.Close"(error in=w551) -> ()  [unwired: 2 in, 3 out]
    }
    frame "Development System" {
    }
  }
  n266 = Close File(refnum=w19, error in=w16) -> (path=w5:path)  [unwired: 1 out]
  n267 = case "update state file if necessary" shown="False" w1 {
    tunnel: w9 -> [w558 w560]
    tunnel: w8 -> [w557 _]
    tunnel: w7 -> [w556 _]
    tunnel: w6 -> [w555 w559]
    tunnel: w5 -> [w554 _]
    tunnel: [w553 w560] -> w4
    tunnel: [w552 w559] -> w3
    frame False {
      n268 = call-poly <vilib>:"Write Key.vi"("section"=w557, "error in (no error)"=w555, "value"=w554, "key"=w556, "refnum"=w558) -> ("error out"=w552:errorcluster, "refnum out"=w553:T6)  [unwired: 4 in, 1 out]
    }
    frame True {
    }
  }
  n269 = call <vilib>:"Close Config Data.vi"("error in (no error)"=w3, "refnum"=w4) -> ()  [unwired: 8 in, 2 out]
